vi "4-11 图形控件之波形图的使用.vi"() -> ()   [LabVIEW 2018]
panel:
  out "波形图 2":dbl[][](graph)
  in  "dx 2":dbl
  in  "x0 2":dbl
  in  "dx":dbl
  in  "x0":dbl
  out "波形图":cluster{"x0 2":dbl, "dx 2":dbl, dbl[]}[](graph)
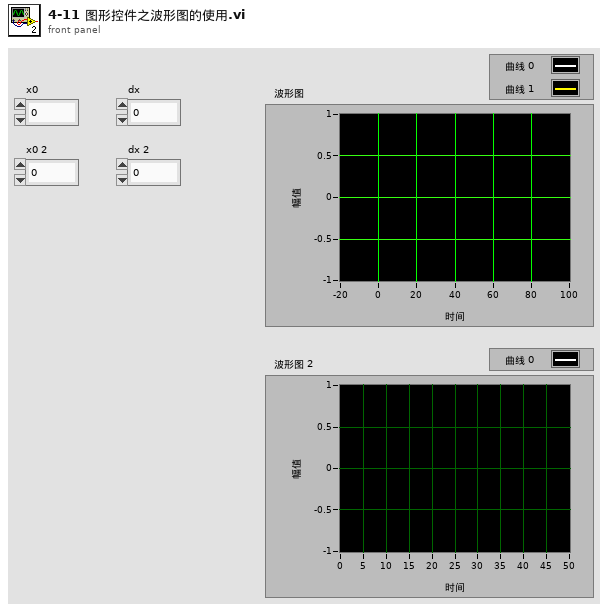
[diagram p1: front panel]
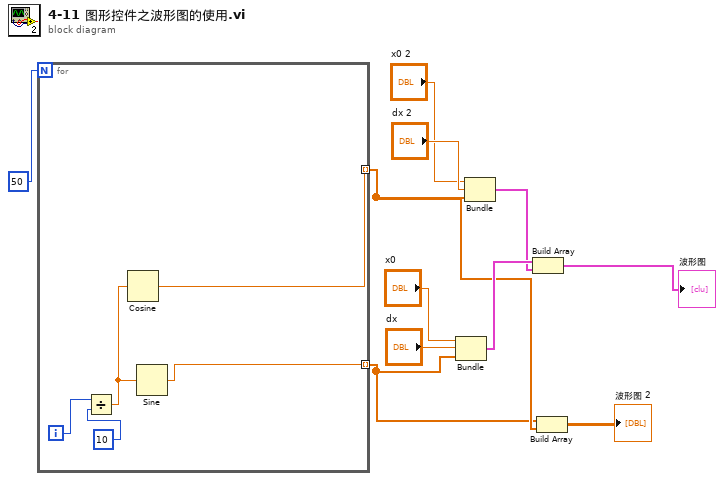
[diagram p0: block diagram]
diagram:
  n1 = for {
    N: 50 -> [_]
    tunnel: [w14] -> w2 mode=indexing
    tunnel: [w12] -> w3 mode=indexing
    i -> [w16]
    n2 = Divide(x=w16, y=10) -> (x/y=w13:dbl)
    n3 = Cosine(x=w13) -> (cos(x)=w12:dbl)
    n4 = Sine(x=w13) -> (sin(x)=w14:dbl)
  }
  n5 = Bundle("x0"="x0", "dx"="dx", w2) -> (w6:cluster{"x0":dbl, "dx":dbl, dbl[]})  [unwired: 1 in]
  n6 = Bundle("x0 2"="x0 2", "dx 2"="dx 2", w3) -> (w5:cluster{"x0 2":dbl, "dx 2":dbl, dbl[]})  [unwired: 1 in]
  n7 = Build Array(w6, w5) -> (→"波形图":cluster{"x0 2":dbl, "dx 2":dbl, dbl[]}[])
  n8 = Build Array(w2, w3) -> (→"波形图 2":dbl[][])
